vi "uti_Ctl_Format.vi"(5 "Write Captions with UserLabels (T)":bool=TRUE, 7 "Write TipStrips with details (T)":bool=TRUE, 8 "error in (no error)":errorcluster, 10 "Channel Config":refnum<class "Config.lvclass">, 11 "Control in":refnum<vi>) -> (0 "error out":errorcluster, 3 "Control out":refnum<vi>)   [LabVIEW 2020, in "UI_Actor.lvlib" / "UI_Actor.lvclass"]
uses:
  UI_Actor.lvclass
  support/Databox.lvlibp/TypesTools/Config/Config.lvclass
  support/Databox.lvlibp/TypesTools/Config/Read System Label.vi
  support/Databox.lvlibp/TypesTools/Config/Read User Label.vi
  support/Databox.lvlibp/TypesTools/Config/Read Unit.vi
  support/Databox.lvlibp/TypesTools/Config/Read Tote bag.vi
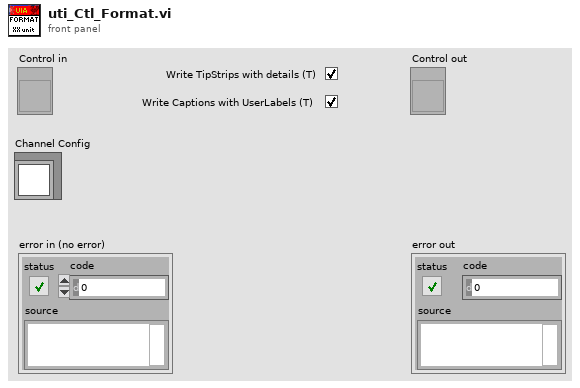
[diagram p1: front panel]
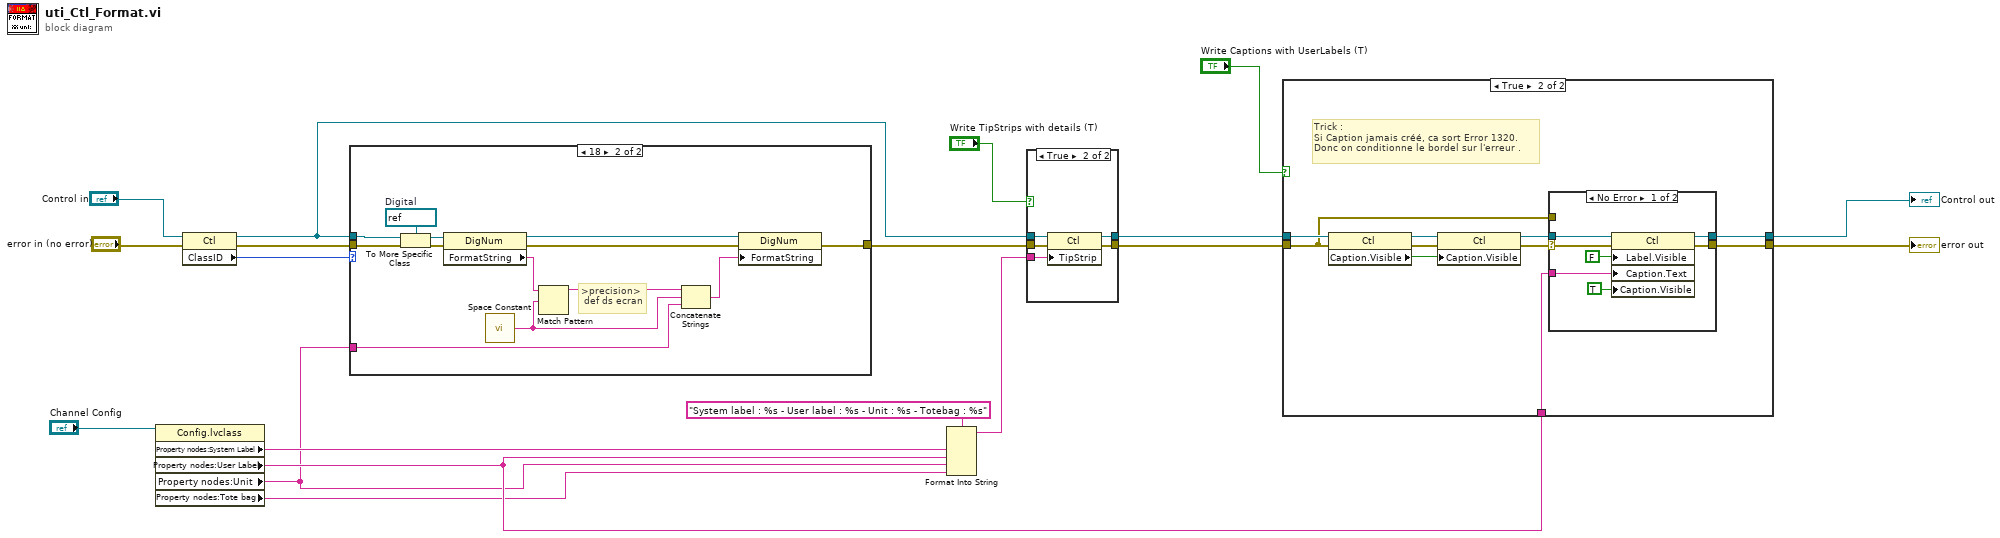
[diagram p0: block diagram]
diagram:
  n1 = property class="Config.lvclass"(reference="Channel Config") -> ("Property nodes:System Label"=w4:string, "Property nodes:User Label"=w3:string, "Property nodes:Unit"=w2:string, "Property nodes:Tote bag"=w1:string)  [unwired: 1 in, 2 out]
  n2 = property class="Ctl"(reference="Control in", error in="error in (no error)") -> (reference out=w14:refnum<vi>, error out=w17:errorcluster, "ClassID"=w16:u32)
  n3 = case shown="18" w16 {
    tunnel: w17 -> [w20 w24]
    tunnel: w14 -> [_ w23]
    tunnel: [w20 w22] -> w15
    tunnel: w2 -> [_ w21]
    frame 0, Default {
    }
    frame 18 {
      w25 = refnum<vi> refnum  # Digital
      # ">precision>\n def ds ecran"
      n4 = To More Specific Class(target class=w25, reference=w23, error in=w24) -> (specific class reference=w27:refnum<vi>, error out=w28:errorcluster)
      n5 = property class="DigNum"(reference=w27, error in=w28) -> (reference out=w29:refnum<vi>, error out=w30:errorcluster, "FormatString"=w31:string)
      n6 = call <vilib>:"Space Constant.vi"() -> ("String"=w33:string)
      n7 = Match Pattern(string=w31, regular expression=w33) -> (before substring=w32:string)  [unwired: 1 in, 3 out]
      n8 = Concatenate Strings(w32, w33, w21) -> (w26:string)
      n9 = property class="DigNum"(reference=w29, error in=w30, "FormatString"=w26) -> (error out=w22:errorcluster)  [unwired: 1 out]
    }
  }
  n10 = Format Into String(format string="System label : %s - User label : %s - Unit : %s - Totebag : %s", w4, w3, w2, w1) -> (resulting string=w12:string)  [unwired: 2 in, 1 out]
  n11 = case shown="True" "Write TipStrips with details (T)" {
    tunnel: w15 -> [w35 w40]
    tunnel: w14 -> [w34 w39]
    tunnel: w12 -> [_ w38]
    tunnel: [w34 w37] -> w9
    tunnel: [w35 w36] -> w8
    frame False {
    }
    frame True {
      n12 = property class="Ctl"(reference=w39, error in=w40, "TipStrip"=w38) -> (reference out=w37:refnum<vi>, error out=w36:errorcluster)
    }
  }
  n13 = case shown="True" "Write Captions with UserLabels (T)" {
    tunnel: w3 -> [_ w52]
    tunnel: [w41 w51] -> w11
    tunnel: [w42 w50] -> w10
    tunnel: w9 -> [w42 w49]
    tunnel: w8 -> [w41 w48]
    frame False {
    }
    frame True {
      # "Trick :\nSi Caption jamais créé, ca sort Error 1320.\nDonc on conditionne le bordel sur l'erreur ."
      n14 = property class="Ctl"(reference=w49, error in=w48) -> (reference out=w47:refnum<vi>, error out=w46:errorcluster, "Caption.Visible"=w43:bool)
      n15 = property class="Ctl"(reference=w47, error in=w46, "Caption.Visible"=w43) -> (reference out=w44:refnum<vi>, error out=w45:errorcluster)
      n16 = case shown="No Error" w45 {
        selector: w45 -> [w53 _]
        tunnel: w52 -> [w58 _]
        tunnel: [w56 w60] -> w51
        tunnel: [w55 w61] -> w50
        tunnel: w44 -> [w54 w61]
        tunnel: w48 -> [_ w60]
        frame No Error {
          n17 = property class="Ctl"(reference=w54, error in=w53, "Label.Visible"=FALSE, "Caption.Text"=w58, "Caption.Visible"=TRUE) -> (reference out=w55:refnum<vi>, error out=w56:errorcluster)
        }
        frame Error {
        }
      }
    }
  }
  "error out" <- w11
  "Control out" <- w10
